vi "SA_MKR_FUNC.vi"(0 "Session In":refnum<visa-resource-name>="TCPIP0::K-N90X0A-00005.local::inst0::INSTR", 1 "Timeout":u32=3000, 2 "RO(T)":bool, 11 "error in":errorcluster {"code" format="%.0x"}, 12 "Span (kHz)":dbl=200000.0, 13 "MKR FUNC":u16(ring) items=["Noise", "Band Power", "Band Interval", "MKR FUNC OFF"]) -> (4 "Session Out":refnum<visa-resource-name>, 8 "Span Out(kHz)":dbl, 14 "FUNC OUT":string, 15 "error out":errorcluster {"code" format="%.0x"})   [LabVIEW 2018]
doc: "N9010 MKR FUNCTION"
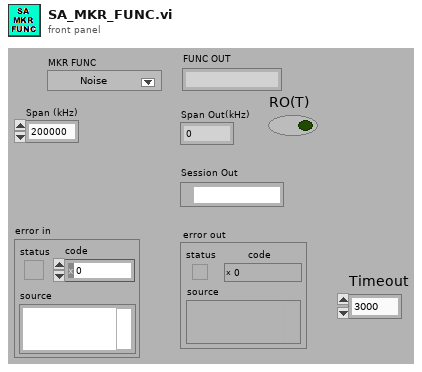
[diagram p1: front panel]
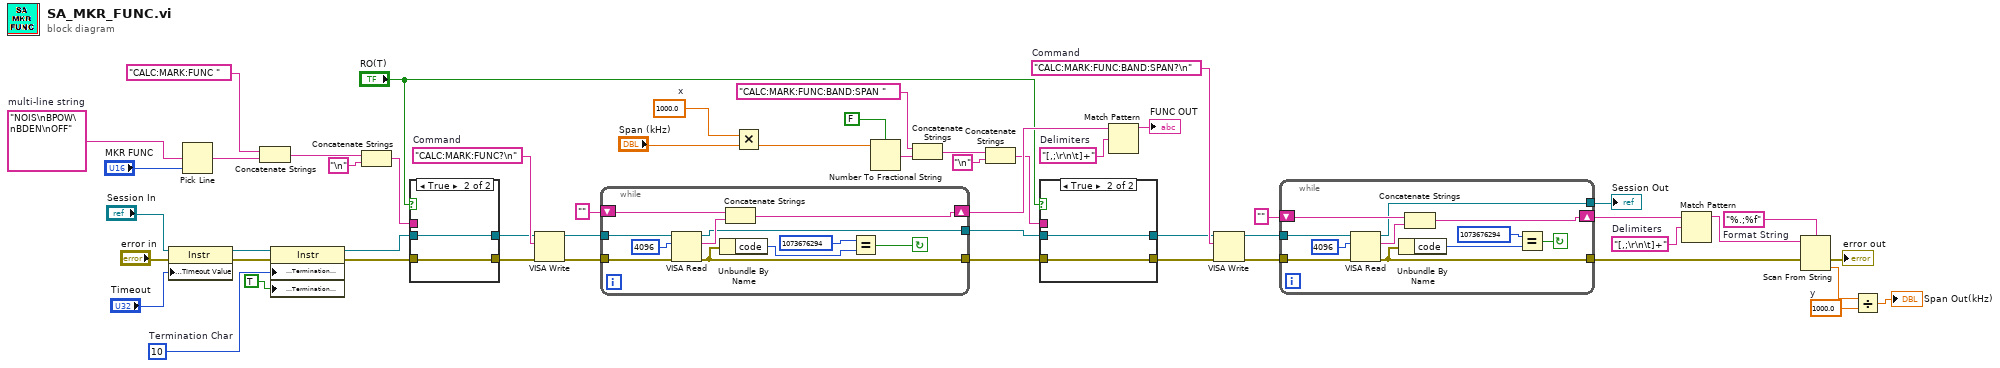
[diagram p0: block diagram]
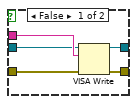
[diagram p2: hidden frame]
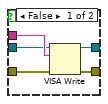
[diagram p3: hidden frame]
diagram:
  w1 = 1000.0  # y
  w4 = 1000.0  # x
  w9 = "NOIS\nBPOW\nBDEN\nOFF"  # multi-line string
  w15 = "[,;\r\n\t]+"  # Delimiters
  w17 = "%.;%f"  # Format String
  w20 = "CALC:MARK:FUNC:BAND:SPAN?\n"  # Command
  w32 = "[,;\r\n\t]+"  # Delimiters
  w34 = "CALC:MARK:FUNC?\n"  # Command
  w46 = u8 10  # Termination Char
  n1 = property class="Instr"(reference="Session In", error in="error in", "General Settings:Timeout Value"="Timeout") -> (reference out=w45:refnum<visa-resource-name>, error out=w48:errorcluster)
  n2 = Pick Line(multi-line string=w9, line index="MKR FUNC") -> (output string=w8:string)  [unwired: 1 in]
  n3 = Concatenate Strings("CALC:MARK:FUNC " ("staticText"), w8) -> (w40:string)
  n4 = property class="Instr"(reference=w45, error in=w48, "Message Based Settings:Termination Character"=w46, "Message Based Settings:Termination Character Enable"=TRUE ("enable")) -> (reference out=w14:refnum<visa-resource-name>, error out=w47:errorcluster)
  n5 = Concatenate Strings(w40, "\n" ("StaticText")) -> (w41:string)
  n6 = case shown="True" "RO(T)" {
    tunnel: w47 -> [w58 w60]
    tunnel: [w57 w60] -> w42
    tunnel: w41 -> [w56 _]
    tunnel: w14 -> [w55 w59]
    tunnel: [w54 w59] -> w13
    frame False {
      n7 = VISA Write(VISA resource name=w55, write buffer=w56, error in (no error)=w58) -> (VISA resource name out=w54:refnum<visa-resource-name>, error out=w57:errorcluster)  [unwired: 1 out]
    }
    frame True {
    }
  }
  n8 = VISA Write(VISA resource name=w13, write buffer=w34, error in (no error)=w42) -> (VISA resource name out=w38:refnum<visa-resource-name>, error out=w37:errorcluster)  [unwired: 1 out]
  n9 = while {
    tunnel: w38 -> [w68]
    shift-right: [w62] -> w31
    shift-left: "" -> [w67]
    tunnel: w37 -> [w65]
    tunnel: [w64] -> w36
    tunnel: [w61] -> w12
    stop <- w63 continue-if-true
    n10 = VISA Read(VISA resource name=w68, byte count=u32 4096 ("byte count (0)"), error in (no error)=w65) -> (VISA resource name out=w61:refnum<visa-resource-name>, read buffer=w66:string, error out=w64:errorcluster)  [unwired: 1 out]
    n11 = Unbundle By Name(w64) -> ("code"=w70:i32)
    n12 = Concatenate Strings(w67, w66) -> (w62:string)
    n13 = Equal?(x=1073676294, y=w70) -> (x = y?=w63:bool)
  }
  n14 = Multiply(x=w4, y="Span (kHz)") -> (x*y=w5:dbl)
  n15 = Number To Fractional String(use system decimal point (T)=FALSE, number=w5) -> (F-format string=w30:string)  [unwired: 2 in]
  n16 = Concatenate Strings("CALC:MARK:FUNC:BAND:SPAN " ("staticText"), w30) -> (w26:string)
  n17 = Concatenate Strings(w26, "\n" ("StaticText")) -> (w27:string)
  n18 = case shown="True" "RO(T)" {
    tunnel: w36 -> [w76 w77]
    tunnel: [w75 w77] -> w28
    tunnel: w27 -> [w74 _]
    tunnel: w12 -> [w73 w78]
    tunnel: [w72 w78] -> w11
    frame False {
      n19 = VISA Write(VISA resource name=w73, write buffer=w74, error in (no error)=w76) -> (VISA resource name out=w72:refnum<visa-resource-name>, error out=w75:errorcluster)  [unwired: 1 out]
    }
    frame True {
    }
  }
  n20 = Match Pattern(string=w31, regular expression=w32) -> (before substring=→"FUNC OUT":string)  [unwired: 4 out]
  n21 = VISA Write(VISA resource name=w11, write buffer=w20, error in (no error)=w28) -> (VISA resource name out=w24:refnum<visa-resource-name>, error out=w23:errorcluster)  [unwired: 1 out]
  n22 = while {
    tunnel: w24 -> [w86]
    shift-right: [w80] -> w19
    shift-left: "" -> [w85]
    tunnel: w23 -> [w83]
    tunnel: [w82] -> w22
    tunnel: [w79] -> w10
    stop <- w81 continue-if-true
    n23 = VISA Read(VISA resource name=w86, byte count=u32 4096 ("byte count (0)"), error in (no error)=w83) -> (VISA resource name out=w79:refnum<visa-resource-name>, read buffer=w84:string, error out=w82:errorcluster)  [unwired: 1 out]
    n24 = Unbundle By Name(w82) -> ("code"=w88:i32)
    n25 = Concatenate Strings(w85, w84) -> (w80:string)
    n26 = Equal?(x=1073676294, y=w88) -> (x = y?=w81:bool)
  }
  "Session Out" <- w10
  n27 = Match Pattern(string=w19, regular expression=w15) -> (before substring=w18:string)  [unwired: 1 in, 3 out]
  n28 = Scan From String(format string=w17, input string=w18, error in=w22) -> (error out=→"error out":errorcluster, output 1=w2:dbl)  [unwired: 2 in, 2 out]
  n29 = Divide(x=w2, y=w1) -> (x/y=→"Span Out(kHz)":dbl)
